vi "ExecuteTactic.vi"(0 "object in":refnum<class "Tactic_v2.lvclass">, 2 "Robot in":refnum<class "Robot.lvclass">, 4 "GameRef":refnum<data-value>, 5 "error in (no error)":errorcluster) -> (14 "object out":refnum<class "Tactic_v2.lvclass">, 16 "Robot out":refnum<class "Robot.lvclass">, 19 "error out":errorcluster)   [LabVIEW 2023, in "Tactic_v2.lvclass"]
uses:
  Tactic_v2.lvclass
  Game_class/Game.lvclass
  Robot_class/Robot.lvclass
  NewSkills/Skill_v2_class/Skill_v2.lvclass
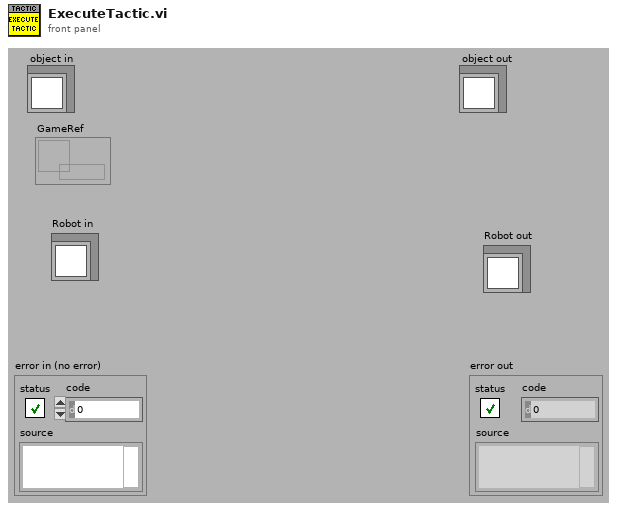
[diagram p1: front panel]
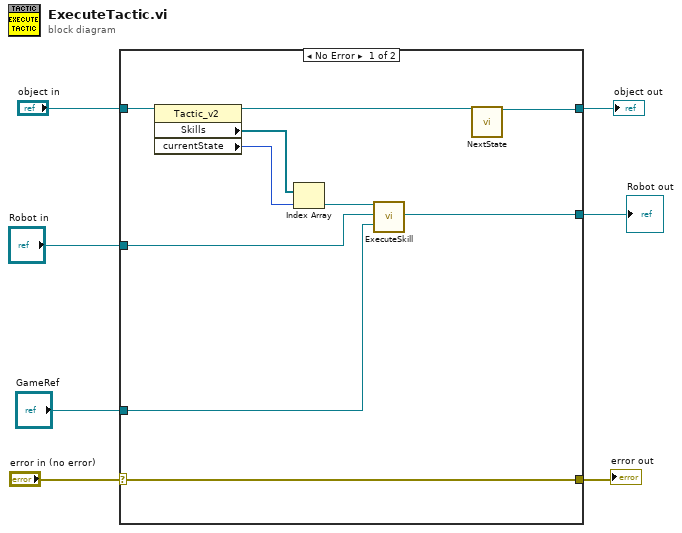
[diagram p0: block diagram]
diagram:
  n1 = case shown="No Error" "error in (no error)" {
    selector: "error in (no error)" -> [w17 w20]
    tunnel: [w17 w20] -> w6
    tunnel: [w8 w19] -> w4
    tunnel: "object in" -> [w16 w19]
    tunnel: "Robot in" -> [w12 w18]
    tunnel: [w11 w18] -> w2
    tunnel: "GameRef" -> [w10 _]
    frame No Error {
      n2 = property class="Tactic_v2"(reference=w16) -> (reference out=w9:refnum<class "Tactic_v2.lvclass">, "Skills"=w15:refnum<class "Skill_v2.lvclass">[], "currentState"=w14:u8)  [unwired: 1 in, 1 out]
      n3 = Index Array(array=w15, index=w14) -> (element=w13:refnum<class "Skill_v2.lvclass">)
      n4 = call-dynamic "ExecuteSkill.vi"("object in"=w13, "Robot in"=w12, "GameRef"=w10) -> ("Robot out"=w11:refnum<class "Robot.lvclass">)  [unwired: 14 in, 2 out]
      n5 = call-dynamic "NextState.vi"("object in"=w9) -> ("object out"=w8:refnum<class "Tactic_v2.lvclass">)  [unwired: 17 in, 1 out]
    }
    frame Error {
    }
  }
  "error out" <- w6
  "object out" <- w4
  "Robot out" <- w2
